vi "AOTF turn off.vi"(3 "error in":errorcluster, 4 "DAQ Setup":enum16{"Test setup", "Microscope"}(ring)=enum."Microscope") -> (10 "error out":errorcluster)   [LabVIEW 2020]
uses:
  <vilib>/DAQmx/write.llb/DAQmx Write (Digital 1D Bool 1Chan 1Samp).vi
  <vilib>/DAQmx/create/channels.llb/DAQmx Create Channel (DO-Digital Output).vi
  <vilib>/DAQmx/miscellaneous.llb/DAQmx Fill In Error Info.vi
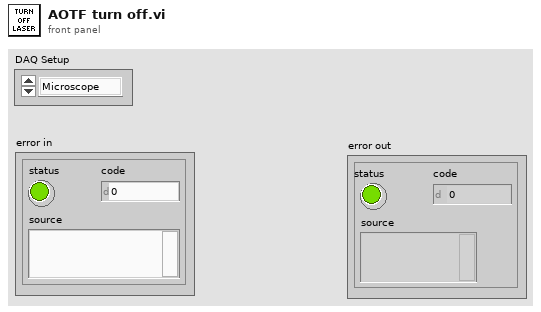
[diagram p1: front panel]
types:
  T1 = typedef "DAQ_channel_typedef.ctl" = cluster{"CO.Pulse.Term":tag, "Voice coil analog output":tag, "counter":tag, "CO.Pulse.Term 2":tag, "AOTF lines":tag, "counter 2":tag, "CO.Pulse.Term 3":tag, "counter 3":tag}
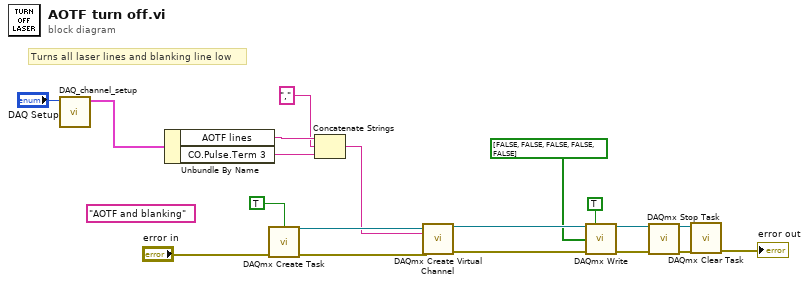
[diagram p0: block diagram]
diagram:
  (unwired) "AOTF and blanking" ("new task name")
  # "Turns all laser lines and blanking line low"
  n1 = call "DAQ_channel_setup.vi"("Text Ring"="DAQ Setup") -> ("DAQ channels OUT"=w8:T1)  [unwired: 10 in]
  n2 = Unbundle By Name(w8) -> ("AOTF lines"=w5:tag, "CO.Pulse.Term 3"=w4:tag)
  n3 = call <vilib>:"DAQmx Create Task.vi"("auto cleanup"=TRUE, "error in"="error in") -> ("task out"=w19:refnum<k21>, "error out"=w18:errorcluster)  [unwired: 12 in]
  n4 = Concatenate Strings(w5, "," ("string"), w4) -> (w2:string)
  n5 = call-poly <vilib>:"DAQmx Create Virtual Channel.vi"("task in"=w19, "lines"=w2, "error in"=w18) -> ("task out"=w17:refnum<k21>, "error out"=w16:errorcluster)  [unwired: 11 in]
  n6 = call-poly <vilib>:"DAQmx Write.vi"("task/channels in"=w17, "auto start"=TRUE, "data"=bool[] [FALSE, FALSE, FALSE, FALSE, FALSE], "error in"=w16) -> ("task out"=w12:refnum<k21>, "error out"=w11:errorcluster)  [unwired: 9 in, 1 out]
  n7 = call <vilib>:"DAQmx Stop Task.vi"("task/channels in"=w12, "error in"=w11) -> ("task out"=w13:refnum<k21>, "error out"=w14:errorcluster)  [unwired: 12 in]
  n8 = call <vilib>:"DAQmx Clear Task.vi"("task in"=w13, "error in"=w14) -> ("error out"=→"error out":errorcluster)  [unwired: 13 in]
